vi "Header_decoder.vi"(0 "header":string) -> (1 "Type":T1=enum."Scope data", 2 "Cargo byte count":u16)   [LabVIEW 2015, in "Hardware.lvlib"]
uses:
  Hardware.lvlib
  Packet type.ctl
panel:
  # "Headers are 4 bytes wide."
  # "MSB: packet type\n01: scope data\n02: ctrl cfg echo"
  # "B1, B2\nCargo packet width"
  # "LSB\nTBD"
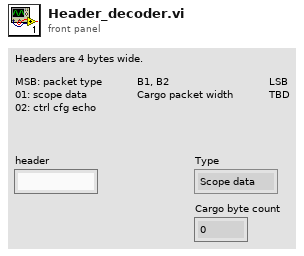
[diagram p1: front panel]
types:
  T1 = typedef "Hardware.lvlib/Packet type.ctl" = enum16{"Null", "Scope data", "Control cfg echo"}
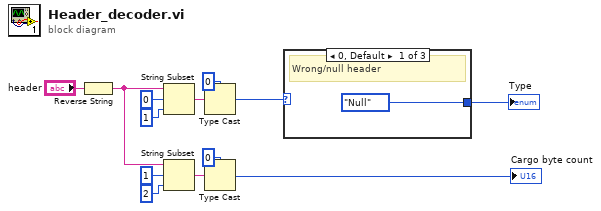
[diagram p0: block diagram]
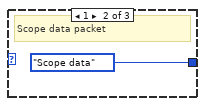
[diagram p2: hidden frame]
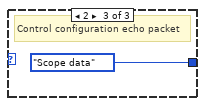
[diagram p3: hidden frame]
diagram:
  n1 = Reverse String(1:"header") -> (0:w2:string)
  n2 = String Subset(string=w2, offset (0)=0, length (rest)=1 ("length (rest)")) -> (substring=w9:string)
  n3 = String Subset(string=w2, offset (0)=1, length (rest)=2 ("length (rest)")) -> (substring=w8:string)
  n4 = Type Cast(type=u8 0 ("length (rest)"), x=w9) -> (*(type *) &x=w3:u8)
  n5 = Type Cast(type=u16 0 ("length (rest)"), x=w8) -> (*(type *) &x=→"Cargo byte count":u16)
  n6 = case shown="0, Default" w3 {
    tunnel: [Packet_type."Null" ("State") Packet_type."Scope data" ("State") Packet_type."Scope data" ("State")] -> w13
    frame 0, Default {
      # "Wrong/null header"
    }
    frame 1 {
      # "Scope data packet"
    }
    frame 2 {
      # "Control configuration echo packet"
    }
  }
  "Type" <- w13
